vi "as2_startLogFile.vi"(4 "error in (no error)":errorcluster, 6 "Path In":path) -> (0 "error out":errorcluster, 2 "Path":path)   [LabVIEW 2009]
uses:
  <vilib>/Utility/file.llb/Write To Spreadsheet File (string).vi
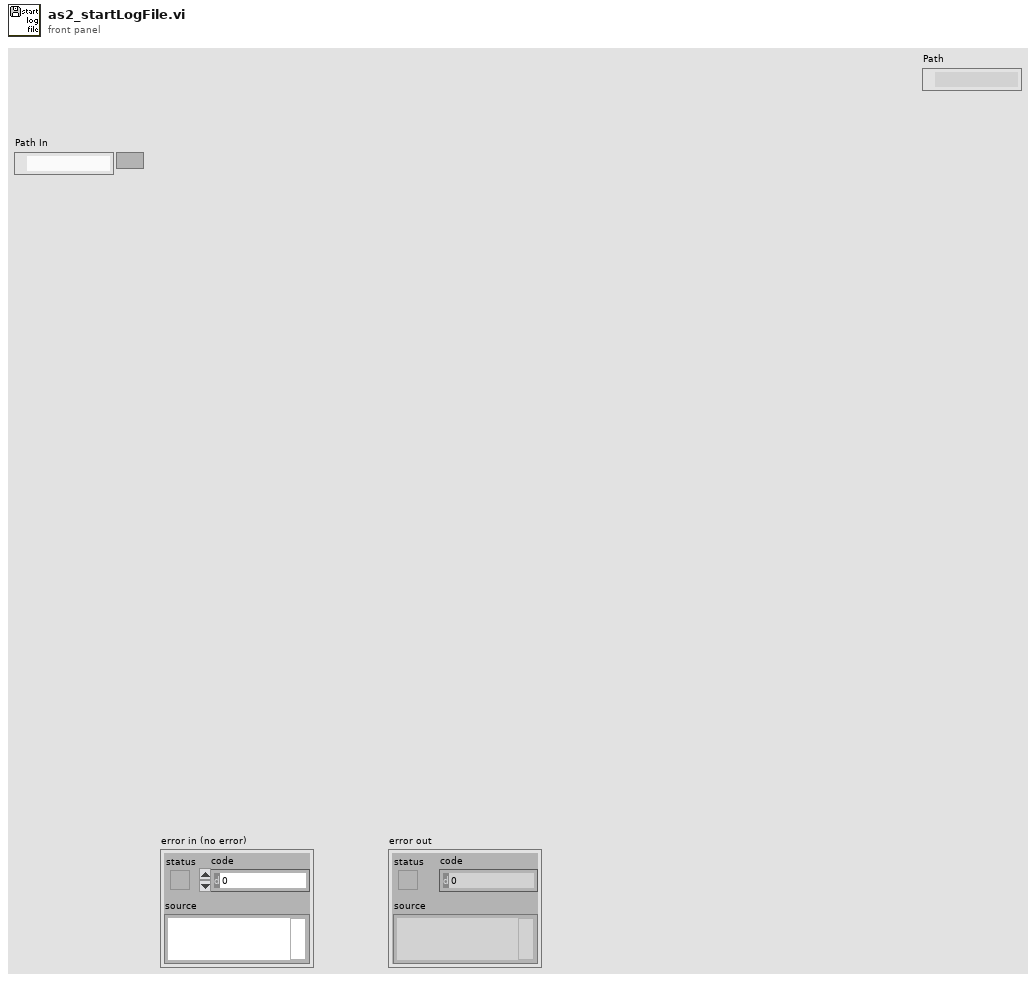
[diagram p1: front panel]
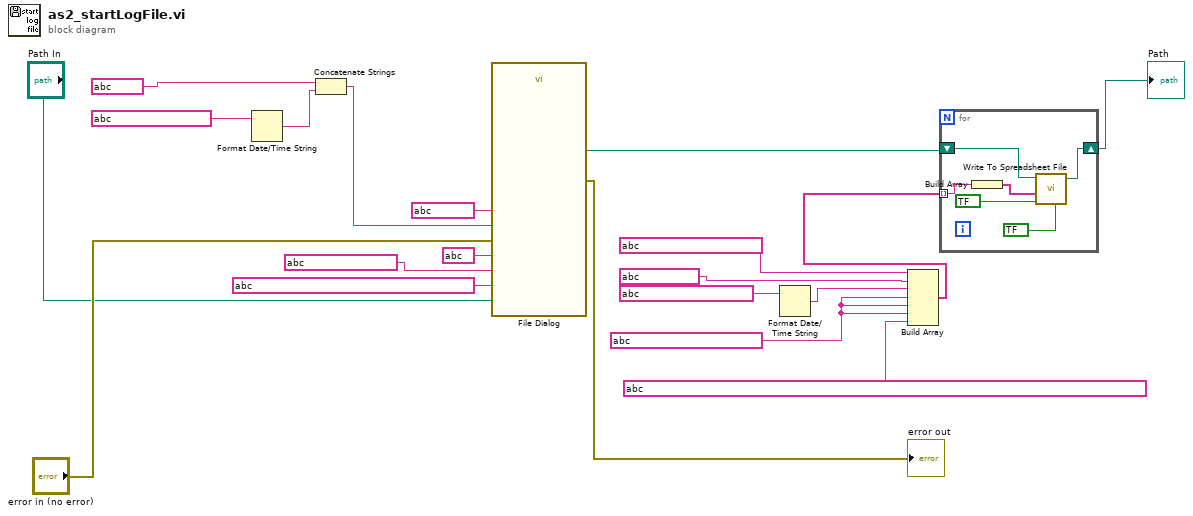
[diagram p0: block diagram]
diagram:
  w1 = string ? ("element")
  n1 = Format Date/Time String(time format string (%c)=string ?) -> (date/time string=w15:string)  [unwired: 2 in]
  n2 = Concatenate Strings(string ?, w15) -> (w14:string)
  n3 = call "File Dialog"("start path"="Path In", "prompt"=string ?, "button label"=string ?, "default name"=w14, "error in"="error in (no error)", "pattern (all files)"=string ?, "pattern label"=string ?) -> ("selected path"=w4:path, "error out"=→"error out":errorcluster)  [unwired: 5 in, 2 out]
  n4 = Format Date/Time String(time format string (%c)=string ?) -> (date/time string=w5:string)  [unwired: 2 in]
  n5 = Build Array(string ?, string ?, w5, w1, w1, w1, string ?) -> (w6:string[])
  n6 = for {
    tunnel: w6 -> [w23] mode=indexing
    shift-right: [w25] -> w3
    shift-left: w4 -> [w24]
    n7 = Build Array(w23) -> (w22:string[])
    n8 = call-poly <vilib>:"Write To Spreadsheet File.vi"("transpose? (no:F)"=bool ?, "append to file? (new file:F)"=bool ?, "1D data"=w22, "file path (dialog if empty)"=w24) -> ("new file path (Not A Path if cancelled)"=w25:path)  [unwired: 4 in]
  }
  "Path" <- w3
